vi "Read FileRef.vi"(8 "error in (no error)":errorcluster, 11 "File Session in":refnum<class "File Session.lvclass">) -> (0 "error out":errorcluster, 2 "FileRef":refnum<file>, 3 "File Session out":refnum<class "File Session.lvclass">)   [LabVIEW 2014, in "File Session.lvclass"]
uses:
  File Session.lvclass
  File Session.lvclass/File Session.ctl
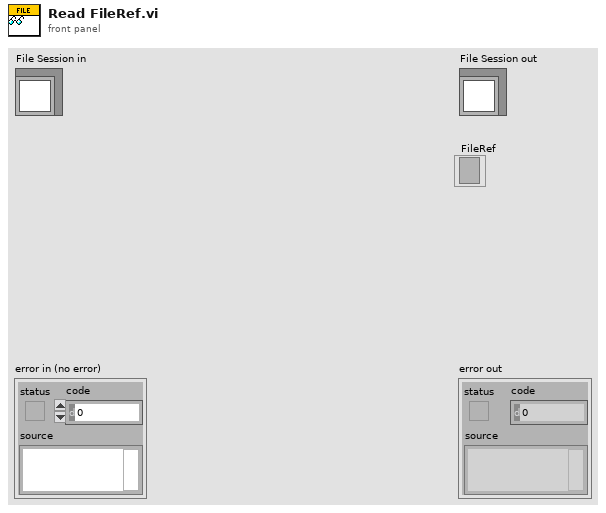
[diagram p1: front panel]
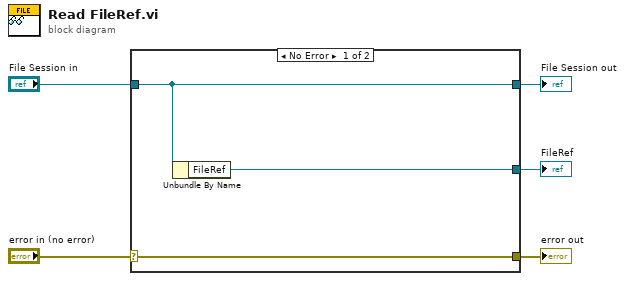
[diagram p0: block diagram]
diagram:
  n1 = case shown="No Error" "error in (no error)" {
    selector: "error in (no error)" -> [w8 w9]
    tunnel: [w8 w9] -> w4
    tunnel: [w7 w10] -> w2
    tunnel: "File Session in" -> [w7 w10]
    tunnel: [w6 _] -> w1
    frame No Error {
      n2 = Unbundle By Name(w7) -> ("FileRef"=w6:refnum<file>)
    }
    frame Error {
    }
  }
  "error out" <- w4
  "File Session out" <- w2
  "FileRef" <- w1
